vi "Sound File to Sound Output.vi"(0 "Volume":dbl(slide)=79.59183673469389 scale=0.0..100.0, 1 "Number of Samples/Iteration":i32=10000, 2 "Device ID":u32, 3 "File Path":path=path "sample.wav") -> ()   [LabVIEW 2013]
doc: "This VI illustrates how to play a sound file continuously, reading the sound file in pieces, and playing each piece at a time."
uses:
  <vilib>/sound2/lvsound2.llb/Sampling Mode.ctl
  <vilib>/sound2/lvsound2.llb/Sound File Info (path).vi
  <vilib>/sound2/lvsound2.llb/Sound File Read Open.vi
  <vilib>/sound2/lvsound2.llb/Sound File Read (DBL).vi
  <vilib>/sound2/lvsound2.llb/Sound Output Set Volume (Single).vi
  <vilib>/sound2/lvsound2.llb/Sound Output Write (DBL).vi
panel:
  out "Loop Index":i32
  in  "stop":bool
  # "This VI plays a sound file continuously, reading the sound file in pieces, and playing each piece at a time.\n\nInstructions to execute the VI:  \n1.  Specify the path for a valid WAV file.\n2.  Specify the Device ID and the Number of samples to read per iteration.\n3.  Run the VI.\n4.  Use the volume slider to dynamically change the volume of the sound played."
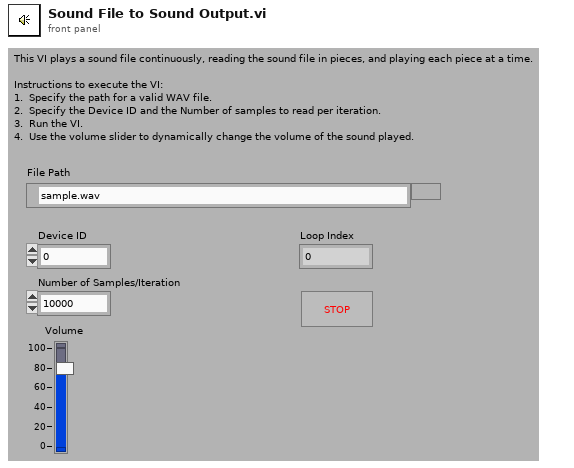
[diagram p1: front panel]
types:
  T1 = typedef "Sampling Mode.ctl" = i32
  T2 = typedef "Sound Data Format.ctl" = cluster{"sample rate (S/s)":dbl, "number of channels":i32, "bits per sample":i32}
  T3 = typedef "Sound File Refnum.ctl" = refnum<file>
  T4 = typedef "Sound Output Task ID.ctl" = u32
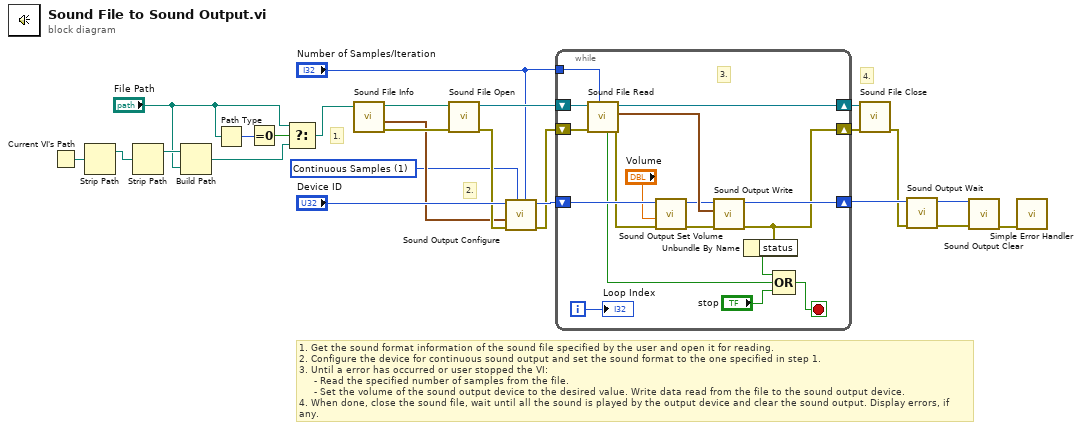
[diagram p0: block diagram]
diagram:
  w10 = T1 1 items=["Finite Samples", "Continuous Samples"] ("sample mode")
  # "4."
  # "2."
  # "1."
  # "1. Get the sound format information of the sound file specified by the user and open it for reading.\n2. Configure the device for continuous sound output and set the sound format to the one specified in step 1.\n3. Until a error has occurred or user stopped the VI:\n    \t- Read the specified number of samples from the file.\n\t    - Set the volume of the sound output device to the desired value. Write data read from the file to the sound output device.\n4. When done, close the sound file, wait until all the sound is played by the output device and clear the sound output. Display errors, if any."
  n1 = Current VI's Path() -> (path=w5:path)
  n2 = Strip Path(path=w5) -> (stripped path=w4:path)  [unwired: 1 out]
  n3 = Strip Path(path=w4) -> (stripped path=w3:path)  [unwired: 1 out]
  n4 = Build Path(base path=w3, name or relative path="File Path") -> (appended path=w6:path)
  n5 = Path Type(1:"File Path") -> (0:w8:i16)
  n6 = Equal To 0?(x=w8) -> (x = 0?=w7:bool)
  n7 = Select(t="File Path", s=w7, f=w6) -> (s? t:f=w2:path)
  n8 = call-poly <vilib>:"Sound File Info.vi"("path"=w2) -> ("error out"=w20:errorcluster, "sound format"=w12:T2, "path out"=w13:path)  [unwired: 7 in, 1 out]
  n9 = call-poly <vilib>:"Sound File Open.vi"("error in (no error)"=w20, "path"=w13) -> ("error out"=w19:errorcluster, "sound file refnum"=w21:T3)  [unwired: 8 in]
  n10 = call <vilib>:"Sound Output Configure.vi"("number of samples/ch"="Number of Samples/Iteration", "sample mode"=w10, "error in (no error)"=w19, "sound format"=w12, "device ID"="Device ID") -> ("error out"=w18:errorcluster, "task ID"=w25:T4)  [unwired: 5 in]
  n11 = while {
    shift-right: [w29] -> w22
    shift-left: w18 -> [w41]
    tunnel: "Number of Samples/Iteration" -> [w28]
    shift-right: [w42] -> w16
    shift-left: w25 -> [w36]
    shift-right: [w37] -> w23
    shift-left: w21 -> [w40]
    i -> [w38]
    stop <- w30 stop-if-true
    # "3."
    n12 = call-poly <vilib>:"Sound File Read.vi"("number of samples/ch (-1: all)"=w28, "error in (no error)"=w41, "sound file refnum"=w40) -> ("error out"=w34:errorcluster, "data"=w39:waveform(dbl)[], "sound file refnum out"=w37:T3, "end of file?"=w31:bool)  [unwired: 4 in, 1 out]
    n13 = call-poly <vilib>:"Sound Output Set Volume.vi"("error in (no error)"=w34, "volume"="Volume", "task ID"=w36) -> ("error out"=w33:errorcluster, "task ID out"=w35:T4)  [unwired: 7 in]
    n14 = call-poly <vilib>:"Sound Output Write.vi"("error in (no error)"=w33, "data"=w39, "task ID"=w35) -> ("error out"=w29:errorcluster, "task ID out"=w42:T4)  [unwired: 7 in]
    n15 = Unbundle By Name(w29) -> ("status"=w27:bool)
    n16 = Compound Arithmetic op=OR(w27, w31, "stop") -> (w30:bool)
    "Loop Index" <- w38
  }
  n17 = call <vilib>:"Sound File Close.vi"("error in (no error)"=w22, "sound file refnum"=w23) -> ("error out"=w15:errorcluster)  [unwired: 9 in]
  n18 = call <vilib>:"Sound Output Wait.vi"("error in (no error)"=w15, "task ID"=w16) -> ("error out"=w14:errorcluster, "task ID out"=w17:T4)  [unwired: 8 in]
  n19 = call <vilib>:"Sound Output Clear.vi"("error in (no error)"=w14, "task ID"=w17) -> ("error out"=w9:errorcluster)  [unwired: 9 in]
  n20 = call <vilib>:"Simple Error Handler.vi"("error in (no error)"=w9) -> ()  [unwired: 4 in, 5 out]
